vi "Datasheet Statistics.vi"(6 "Connection Refnum":T3, 8 "error in (no error)":errorcluster, 9 "Grouped Results":cluster{"Result Group":T1[]}[](array[cluster]), 10 "sxTemplateId":string, 11 "Parameters":T2) -> (0 "error out":errorcluster, 3 "report":path)   [LabVIEW 2011]
uses:
  SI.LIB/ODBC/SQL Controls/Connection Refnum.ctl
  Addons/internet/utils/keyedarr.llb/Keyed Array.ctl
  www/cgi-bin/_cgi-lib/TDM_INDEX Record.ctl
  Addons/internet/utils/strutil.llb/Case Matching.ctl
  Datasheet Analysis Parameters.ctl
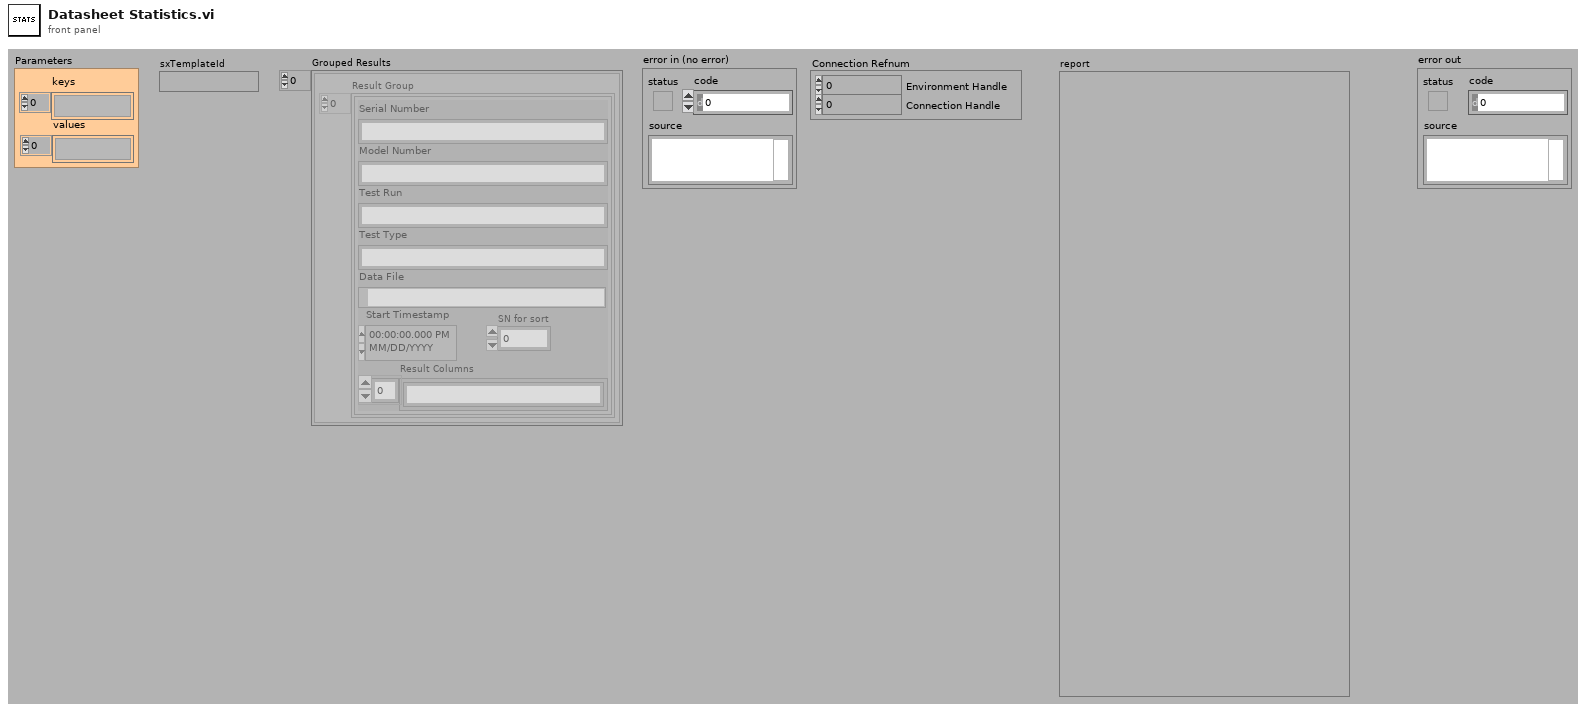
[diagram p1: front panel]
types:
  T1 = typedef "TDM_INDEX Record.ctl" = cluster{"Model Number":string, "SN for sort":i32, "Test Type":string, "Test Run":string, "Serial Number":string, "Start Timestamp":timestamp, "Data File":path, "Result Columns":string[]}
  T2 = typedef "Keyed Array.ctl" = cluster{"keys":string[], "values":string[]}
  T3 = typedef "Connection Refnum.ctl" = cluster{"Environment Handle":i32, "Connection Handle":i32}
  T4 = typedef "Datasheet Analysis Parameters.ctl" = cluster{"Test Type":string, "Parameter":string, "Sxx Format":string, "PIM Unit":string, "Start Frequency":dbl, "Stop Frequency":dbl, "Sort Property":string, "Show Raw?":bool, "Bin format":string, "Bin Type":string, "Bin_var":string}
  T5 = typedef "Case Matching.ctl" = enum16{"a != A", "a == A", "system"}
  T6 = typedef "Statistics Data.ctl" = cluster{"Table":T7[], "Frequencies":dbl[]}
  T7 = typedef "CGI SimpleStat Results.ctl" = cluster{"Model Number":string, "Serial Number for Sort":i32, "Serial Number":string, "Time Stamp":timestamp, "Channel Data":dbl[], "Test Status":string, "OperatorID":string, "Frequency Data":dbl[], "RunID":string, "Sort Property Value":string}
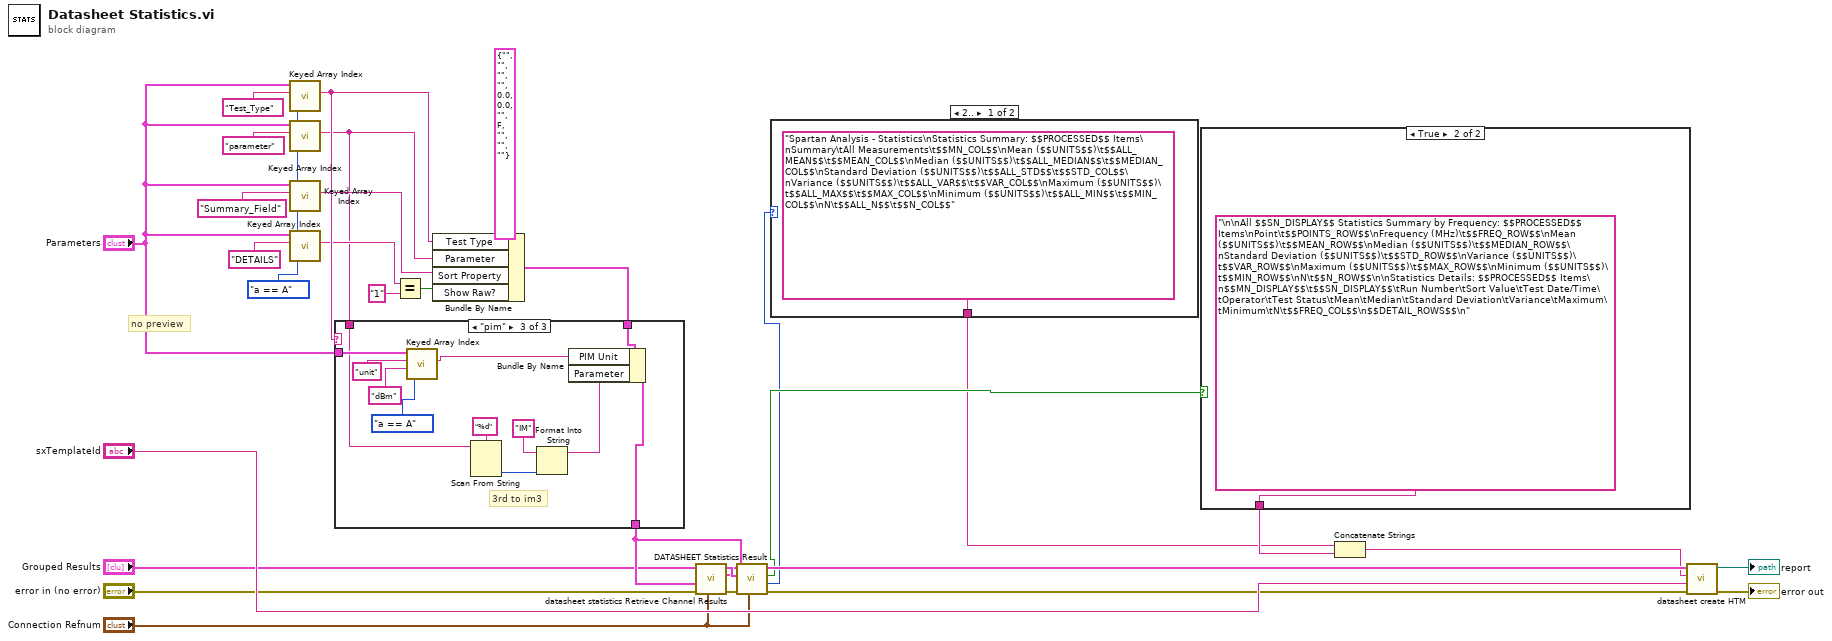
[diagram p0: block diagram]
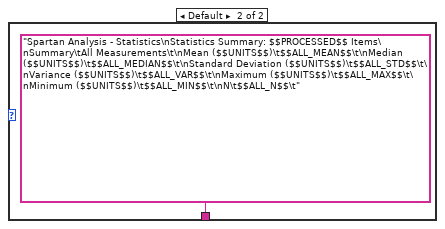
[diagram p2: hidden frame]
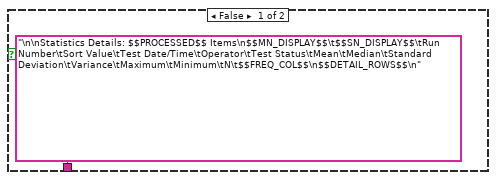
[diagram p3: hidden frame]
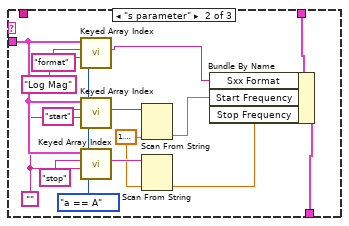
[diagram p5: hidden frame]
diagram:
  w8 = Case_Matching."a == A" ("case matching (sensitive)")
  # "no preview"
  n1 = call "Keyed Array Index.vi"("case matching (sensitive)"=w8, "key"="Test_Type" ("format string"), "array in"="Parameters") -> ("value"=w19:string)  [unwired: 1 in, 3 out]
  n2 = call "Keyed Array Index.vi"("case matching (sensitive)"=w8, "key"="parameter" ("format string"), "array in"="Parameters") -> ("value"=w7:string)  [unwired: 1 in, 3 out]
  n3 = call "Keyed Array Index.vi"("case matching (sensitive)"=w8, "key"="Summary_Field" ("format string"), "array in"="Parameters") -> ("value"=w12:string)  [unwired: 1 in, 3 out]
  n4 = call "Keyed Array Index.vi"("case matching (sensitive)"=w8, "key"="DETAILS" ("format string"), "array in"="Parameters") -> ("value"=w16:string)  [unwired: 1 in, 3 out]
  n5 = Equal?(x=w16, y="1" ("format string")) -> (x = y?=w17:bool)
  n6 = Bundle By Name(cluster=T4 {"Test Type"="", "Parameter"="", "Sxx Format"="", "PIM Unit"="", "Start Frequency"=0.0, "Stop Frequency"=0.0, "Sort Property"="", "Show Raw?"=FALSE, "Bin format"="", "Bin Type"="", "Bin_var"=""} ("Test Parameters"), "Test Type"=w19, "Parameter"=w7, "Sort Property"=w12, "Show Raw?"=w17) -> (w20:T4)
  n7 = case shown="\"pim\"" w19 {
    tunnel: "Parameters" -> [_ w44 w58]
    tunnel: w20 -> [w31 w43 w57]
    tunnel: [w31 w42 w56] -> w22
    tunnel: w7 -> [_ _ w48]
    frame Default {
    }
    frame "s parameter" {
      w41 = Case_Matching."a == A" ("case matching (sensitive)")
      w33 = 1.1447298858494002
      w38 = ""
      n8 = call "Keyed Array Index.vi"("case matching (sensitive)"=w41, "default value"="Log Mag" ("format string"), "key"="format" ("format string"), "array in"=w44) -> ("value"=w40:string)  [unwired: 3 out]
      n9 = call "Keyed Array Index.vi"("case matching (sensitive)"=w41, "default value"=w38, "key"="start" ("format string"), "array in"=w44) -> ("value"=w36:string)  [unwired: 3 out]
      n10 = call "Keyed Array Index.vi"("case matching (sensitive)"=w41, "default value"=w38, "key"="stop" ("format string"), "array in"=w44) -> ("value"=w34:string)  [unwired: 3 out]
      n11 = Scan From String(input string=w36, default 1=w33) -> (output 1=w35:dbl)  [unwired: 3 in, 3 out]
      n12 = Scan From String(input string=w34, default 1=w33) -> (output 1=w32:dbl)  [unwired: 3 in, 3 out]
      n13 = Bundle By Name(cluster=w43, "Sxx Format"=w40, "Start Frequency"=w35, "Stop Frequency"=w32) -> (w42:T4)
    }
    frame "pim" {
      # "3rd to im3"
      n14 = call "Keyed Array Index.vi"("case matching (sensitive)"=Case_Matching."a == A", "default value"="dBm" ("format string"), "key"="unit" ("format string"), "array in"=w58) -> ("value"=w55:string)  [unwired: 3 out]
      n15 = Scan From String(format string="%d", input string=w48) -> (output 1=w50:i32)  [unwired: 2 in, 4 out]
      n16 = Format Into String(initial string="IM" ("format string"), w50) -> (resulting string=w47:string)  [unwired: 2 in, 1 out]
      n17 = Bundle By Name(cluster=w57, "PIM Unit"=w55, "Parameter"=w47) -> (w56:T4)
    }
  }
  n18 = call "datasheet statistics Retrieve Channel Results.vi"("Connection Refnum"="Connection Refnum", "error in (no error)"="error in (no error)", "Test Parameters"=w22, "Grouped Results"="Grouped Results") -> ("error out"=w21:errorcluster, "Stat Data"=w23:T6)  [unwired: 6 out]
  n19 = call "DATASHEET Statistics Result.vi"("Connection Refnum"="Connection Refnum", "error in (no error)"=w21, "Statistics Results"=w23, "Query Parameters"=w22) -> ("error out"=w27:errorcluster, "columns"=w4:i32, "FORM"=w5:bool, "Keyed Array"=w29:T2)  [unwired: 1 in, 3 out]
  n20 = case shown="2.." w4 {
    tunnel: ["Spartan Analysis - Statistics\nStatistics Summary: $$PROCESSED$$ Items\nSummary\tAll Measurements\t$$MN_COL$$\nMean ($$UNITS$$)\t$$ALL_MEAN$$\t$$MEAN_COL$$\nMedian ($$UNITS$$)\t$$ALL_MEDIAN$$\t$$MEDIAN_COL$$\nStandard Deviation ($$UNITS$$)\t$$ALL_STD$$\t$$STD_COL$$\nVariance ($$UNITS$$)\t$$ALL_VAR$$\t$$VAR_COL$$\nMaximum ($$UNITS$$)\t$$ALL_MAX$$\t$$MAX_COL$$\nMinimum ($$UNITS$$)\t$$ALL_MIN$$\t$$MIN_COL$$\nN\t$$ALL_N$$\t$$N_COL$$" "Spartan Analysis - Statistics\nStatistics Summary: $$PROCESSED$$ Items\nSummary\tAll Measurements\t\nMean ($$UNITS$$)\t$$ALL_MEAN$$\t\nMedian ($$UNITS$$)\t$$ALL_MEDIAN$$\t\nStandard Deviation ($$UNITS$$)\t$$ALL_STD$$\t\nVariance ($$UNITS$$)\t$$ALL_VAR$$\t\nMaximum ($$UNITS$$)\t$$ALL_MAX$$\t\nMinimum ($$UNITS$$)\t$$ALL_MIN$$\t\nN\t$$ALL_N$$\t"] -> w1
    frame 2.. {
    }
    frame Default {
    }
  }
  n21 = case shown="True" w5 {
    tunnel: ["\n\nStatistics Details: $$PROCESSED$$ Items\n$$MN_DISPLAY$$\t$$SN_DISPLAY$$\tRun Number\tSort Value\tTest Date/Time\tOperator\tTest Status\tMean\tMedian\tStandard Deviation\tVariance\tMaximum\tMinimum\tN\t$$FREQ_COL$$\n$$DETAIL_ROWS$$\n" "\n\nAll $$SN_DISPLAY$$ Statistics Summary by Frequency: $$PROCESSED$$ Items\nPoint\t$$POINTS_ROW$$\nFrequency (MHz)\t$$FREQ_ROW$$\nMean ($$UNITS$$)\t$$MEAN_ROW$$\nMedian ($$UNITS$$)\t$$MEDIAN_ROW$$\nStandard Deviation ($$UNITS$$)\t$$STD_ROW$$\nVariance ($$UNITS$$)\t$$VAR_ROW$$\nMaximum ($$UNITS$$)\t$$MAX_ROW$$\nMinimum ($$UNITS$$)\t$$MIN_ROW$$\nN\t$$N_ROW$$\n\nStatistics Details: $$PROCESSED$$ Items\n$$MN_DISPLAY$$\t$$SN_DISPLAY$$\tRun Number\tSort Value\tTest Date/Time\tOperator\tTest Status\tMean\tMedian\tStandard Deviation\tVariance\tMaximum\tMinimum\tN\t$$FREQ_COL$$\n$$DETAIL_ROWS$$\n"] -> w3
    frame False {
    }
    frame True {
    }
  }
  n22 = Concatenate Strings(w1, w3) -> (w2:string)
  n23 = call "datasheet create HTM.vi"("error in (no error)"=w27, "sxTemplateId"="sxTemplateId", "template"=w2, "array out"=w29) -> ("error out"=→"error out":errorcluster, "report"=→"report":path)  [unwired: 6 out]
